vi "Init Events.vi"(8 "error in (no error)":errorcluster, 11 "LV Chat Client in":refnum<class "LV Chat Client.lvclass">) -> (0 "error out":errorcluster, 3 "LV Chat Client out":refnum<class "LV Chat Client.lvclass">)   [LabVIEW 2020, in "LV Chat Client.lvclass"]
uses:
  LV Chat Client.lvclass
  <vilib>/IlluminatedG/lv-stream/Connection State.ctl
  Data Types/User Info.ctl
  Data Types/Message.ctl
  LV Chat Client.lvclass/LV Chat Client.ctl
  <vilib>/IlluminatedG/lv-stream/Stream.lvlib
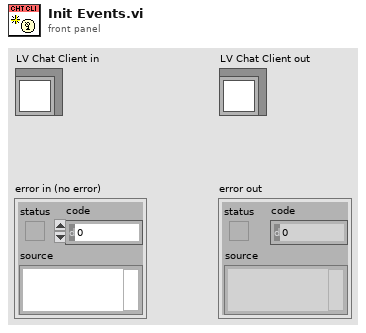
[diagram p1: front panel]
types:
  T1 = typedef "Message.ctl" = cluster{"From":string, "Time":dbl, "Message":string}
  T2 = typedef "User Info.ctl" = cluster{"Name":string}
  T3 = typedef "Stream.lvlib/Connection State.ctl" = enum16{"Connected", "Disconnected"}
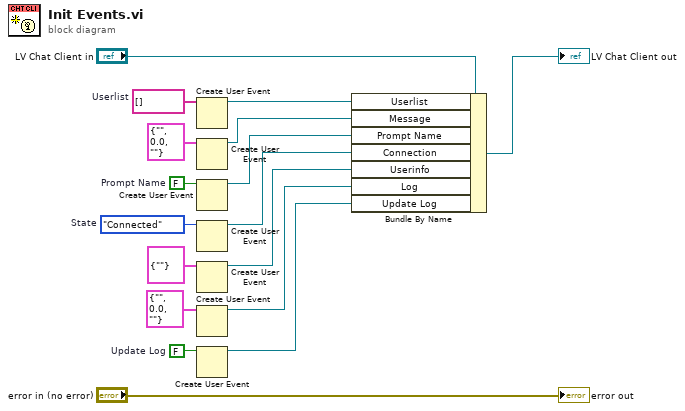
[diagram p0: block diagram]
diagram:
  w2 = FALSE  # Update Log
  w8 = Connection_State."Connected"  # State
  w10 = FALSE  # Prompt Name
  w15 = string[] []  # Userlist
  n1 = Create User Event(user event datatype=w15) -> (user event=w13:refnum<user-event>)  [unwired: 1 in, 1 out]
  n2 = Create User Event(user event datatype=T1 {"From"="", "Time"=0.0, "Message"=""} ("Message")) -> (user event=w11:refnum<user-event>)  [unwired: 1 in, 1 out]
  n3 = Create User Event(user event datatype=w10) -> (user event=w9:refnum<user-event>)  [unwired: 1 in, 1 out]
  n4 = Create User Event(user event datatype=w8) -> (user event=w7:refnum<user-event>)  [unwired: 1 in, 1 out]
  n5 = Create User Event(user event datatype=T2 {"Name"=""} ("User Info")) -> (user event=w5:refnum<user-event>)  [unwired: 1 in, 1 out]
  n6 = Create User Event(user event datatype=T1 {"From"="", "Time"=0.0, "Message"=""} ("Message")) -> (user event=w3:refnum<user-event>)  [unwired: 1 in, 1 out]
  n7 = Create User Event(user event datatype=w2) -> (user event=w1:refnum<user-event>)  [unwired: 1 in, 1 out]
  n8 = Bundle By Name(cluster="LV Chat Client in", "Userlist"=w13, "Message"=w11, "Prompt Name"=w9, "Connection"=w7, "Userinfo"=w5, "Log"=w3, "Update Log"=w1) -> (→"LV Chat Client out":refnum<class "LV Chat Client.lvclass">)
  "error out" <- "error in (no error)"
